vi "element_editor_init_tree.vi"(10 "LUA Specification File":path, 11 "TreeControl in":refnum<vi>) -> ()   [LabVIEW 2019]
uses:
  lib/libSpecValiReader/libSpecValiReader.lvlib
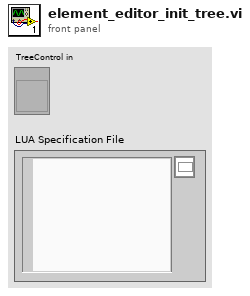
[diagram p1: front panel]
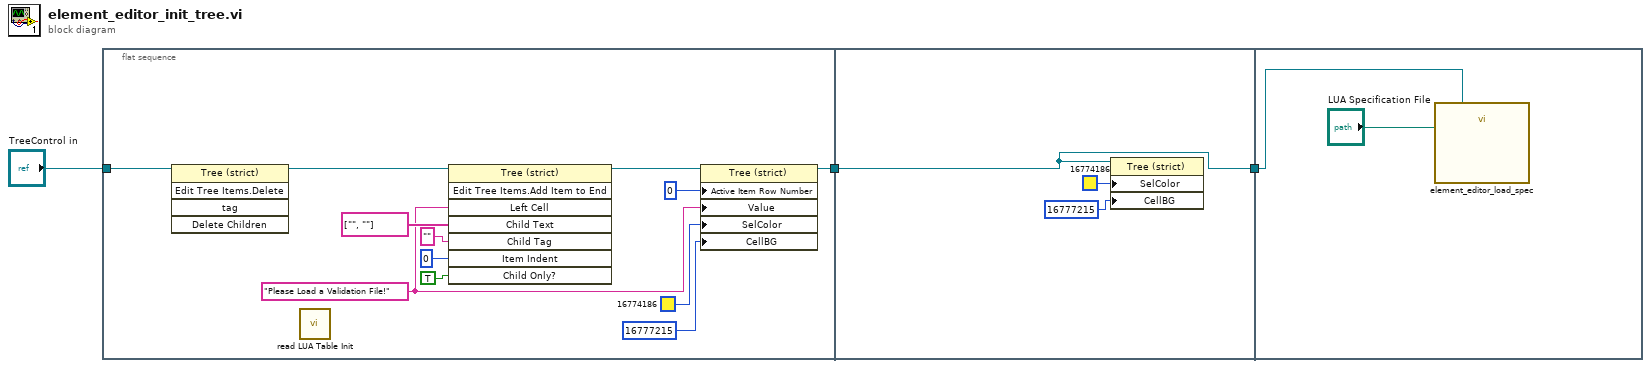
[diagram p0: block diagram]
diagram:
  n1 = flat-sequence {
    tunnel: "TreeControl in" -> [w15]
    tunnel: [w4] -> w3
    tunnel: w3 -> [w18]
    tunnel: [w18] -> w2
    tunnel: w2 -> [w20]
    frame #0 {
      w5 = "Please Load a Validation File!" ("Parent Tag")
      n2 = invoke on="Invoke Node" class="Tree (strict)" method="Edit Tree Items.Delete"(reference=w15) -> (reference out=w7:refnum<vi>)  [unwired: 4 in, 4 out]
      n3 = call "read LUA Table Init.vi"() -> ()  [unwired: 11 in, 1 out]
      n4 = invoke on="Invoke Node" class="Tree (strict)" method="Edit Tree Items.Add Item to End"(reference=w7, "Left Cell"=w5, "Child Text"=string[] ["", ""], "Child Tag"="", "Item Indent"=0 ("New Item Indentation"), "Child Only?"=TRUE) -> (reference out=w6:refnum<vi>)  [unwired: 2 in, 7 out]
      n5 = property on="Property Node" class="Tree (strict)"(reference=w6, "Active Item Row Number"=0 ("Active Item:Row Number"), "Value"=w5, "SelColor"=u32 16774186, "CellBG"=u32 16777215 ("Active Cell:Background Color")) -> (reference out=w4:refnum<vi>)  [unwired: 1 in, 1 out]
    }
    frame #1 {
      n6 = property on="Property Node" class="Tree (strict)"(reference=w18, "SelColor"=u32 16774186, "CellBG"=u32 16777215 ("Active Cell:Background Color")) -> ()  [unwired: 1 in, 2 out]
    }
    frame #2 {
      n7 = call "element_editor_load_spec.vi"("LUA Specification File"="LUA Specification File", "Parameters Tree"=w20) -> ()  [unwired: 8 in, 2 out]
    }
  }
